vi "Alarms.vi"() -> ()   [LabVIEW 2012]
panel:
  out "Time Stamp Control":timestamp format="%<%H:%M:%S%2u\n%d/%m/%Y>T"
  out "sysStat":bool caption="System Status"
  out "senseConn":bool caption="Sensor Connection"
  out "High O2 Level":bool
  out "Altitude":bool
  out "Low O2 Level":bool
  out "CO2 Level":bool
  out "Sensor Error":bool
  out "Calibrate":bool
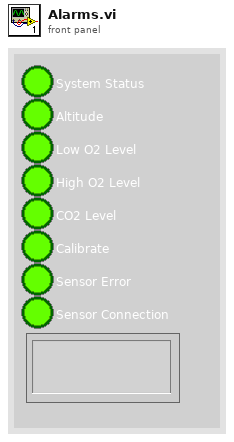
[diagram p1: front panel]
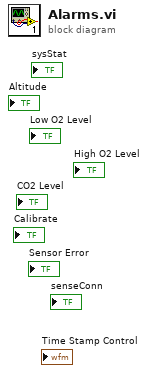
[diagram p0: block diagram]
diagram:
